vi "Reset.vi"(8 "error in (no error)":errorcluster, 11 "ClassIn":refnum<class "NiPxi6733.lvclass">) -> (0 "error out":errorcluster, 3 "ClassOut":refnum<class "NiPxi6733.lvclass">)   [LabVIEW 2014, in "FGenPlugins.lvlib" / "NiPxi6733.lvclass"]
uses:
  NiPxi6733.lvclass
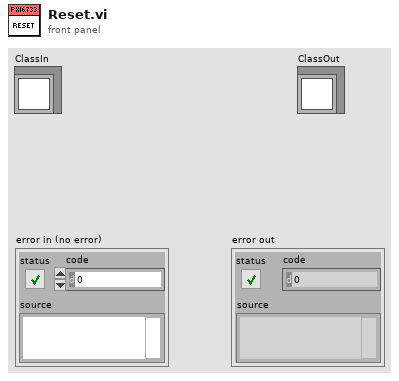
[diagram p1: front panel]
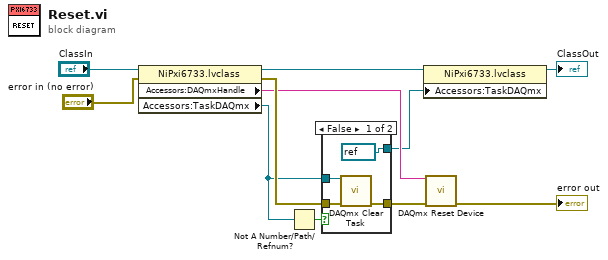
[diagram p0: block diagram]
diagram:
  n1 = property class="NiPxi6733.lvclass"(reference="ClassIn", error in="error in (no error)") -> (reference out=w6:refnum<class "NiPxi6733.lvclass">, error out=w9:errorcluster, "Accessors:DAQmxHandle"=w8:tag, "Accessors:TaskDAQmx"=w3:refnum<k21>)
  n2 = Not A Number/Path/Refnum?(number/path/refnum=w3) -> (NaN/Path/Refnum?=w4:bool)
  n3 = case shown="False" w4 {
    tunnel: w9 -> [w15 w17]
    tunnel: [w14 w17] -> w5
    tunnel: w3 -> [w13 w16]
    tunnel: [refnum<k21> refnum ("Accessors:TaskDAQmx") w16] -> w1
    frame False {
      n4 = call <vilib>:"DAQmx Clear Task.vi"("task in"=w13, "error in"=w15) -> ("error out"=w14:errorcluster)  [unwired: 13 in]
    }
    frame True {
    }
  }
  n5 = property class="NiPxi6733.lvclass"(reference=w6, "Accessors:TaskDAQmx"=w1) -> (reference out=→"ClassOut":refnum<class "NiPxi6733.lvclass">)  [unwired: 1 in, 1 out]
  n6 = call <vilib>:"DAQmx Reset Device.vi"("device in"=w8, "error in"=w5) -> ("error out"=→"error out":errorcluster)  [unwired: 13 in]
